vi "SetTempAndMeasure.vi"() -> ()   [LabVIEW 2009]
uses:
  <instrlib>/BK Precision 91xx Series/BK Precision 91xx Series.lvlib
panel:
  out "error out":errorcluster
  in  "Serial Configuration":T1={"Parity(0:none)"=0, "Baud Rate (9600)"=9600, "Data Bits(8)"=8, "Flow Control(None)"=0, " Stop Bits(1.0)"=10} {"Stop Bits(1.0)" items=["1.0"=10, "1.5"=15, "2.0"=20]; "Flow Control(None)" items=["None", "XON/XOFF", "RTS/CTS", "XON/XOFF & RTS/CTS", "DTR/DSR", "XON/XOFF & DTR/DSR"]; "Data Bits(8)" items=["7"=7, "8"=8]; "Baud Rate (9600)" items=["2400"=2400, "4800"=4800, "9600"=9600, "19200"=19200, "38400"=38400]; "Parity(0:none)" items=["None", "Odd", "Even", "Mark", "Space"]}
  in  "VISA resource name":refnum<visa-resource-name>
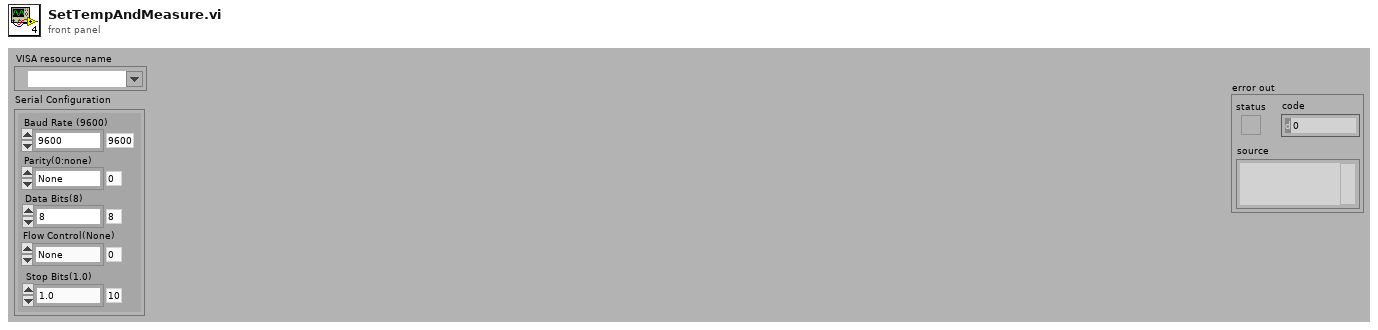
[diagram p1: front panel]
types:
  T1 = cluster{"Parity(0:none)":u16, "Baud Rate (9600)":u16, "Data Bits(8)":u16, "Flow Control(None)":u16, " Stop Bits(1.0)":u16}
  T2 = enum16{"open", "replace", "create", "open or create", "replace or create", "replace or create with confirmation"}
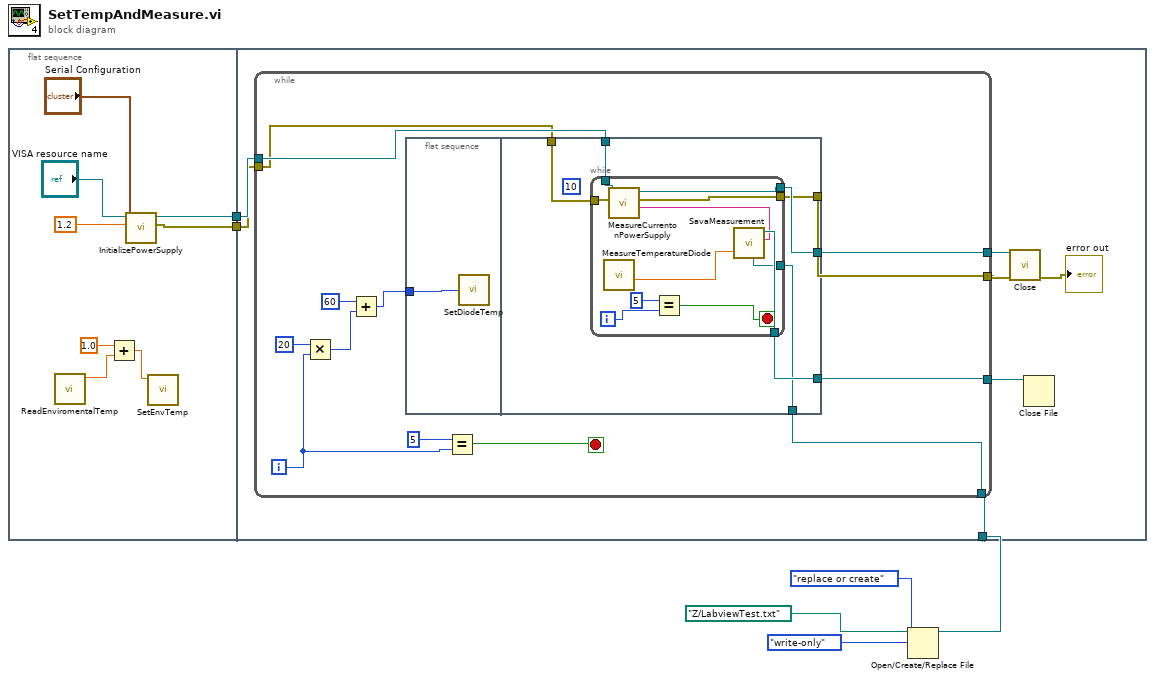
[diagram p0: block diagram]
diagram:
  n1 = flat-sequence {
    tunnel: [w8] -> w2
    tunnel: [w7] -> w1
    tunnel: w3 -> [w17]
    tunnel: w2 -> [w16]
    tunnel: w1 -> [w15]
    frame #0 {
      n2 = call "ReadEnviromentalTemp.vi"() -> ("Probe 1 temperature"=w10:dbl)  [unwired: 10 in, 1 out]
      n3 = Add(x=1.0, y=w10) -> (x+y=w11:dbl)
      n4 = call "InitializePowerSupply.vi"("Serial Configuration"="Serial Configuration", "Manual Range(0.00)"=1.2, "VISA resource name"="VISA resource name") -> ("error out"=w7:errorcluster, "VISA resource name out"=w8:refnum<visa-resource-name>)  [unwired: 7 in]
      n5 = call "SetEnvTemp.vi"("New temperature"=w11) -> ()  [unwired: 10 in, 1 out]
    }
    frame #1 {
      n6 = while {
        tunnel: [w34] -> w20
        tunnel: [w33] -> w19
        tunnel: [w32] -> w18
        tunnel: w17 -> [w31]
        tunnel: w16 -> [w23]
        tunnel: w15 -> [w22]
        i -> [w28]
        stop <- w29 stop-if-true
        n7 = Multiply(x=20, y=w28) -> (x*y=w26:i32)
        n8 = Add(x=60, y=w26) -> (x+y=w24:i32)
        n9 = flat-sequence {
          tunnel: w24 -> [w35]
          tunnel: [w41] -> w34
          tunnel: [w40] -> w33
          tunnel: [w39] -> w32
          tunnel: w31 -> [w38]
          tunnel: w23 -> [w37]
          tunnel: w22 -> [w36]
          frame #0 {
            n10 = call "SetDiodeTemp.vi"(w35) -> ()
          }
          frame #1 {
            (unwired) 10
            n11 = while {
              tunnel: [w52] -> w41
              tunnel: [w51] -> w40
              tunnel: [w50] -> w39
              tunnel: w38 -> [w44]
              tunnel: w37 -> [w43]
              tunnel: w36 -> [w42]
              i -> [w47]
              stop <- w46 stop-if-true
              n12 = call "MeasureTemperatureDiode.vi"() -> ("Celcius"=w49:dbl)  [unwired: 8 in, 3 out]
              n13 = call "MeasureCurrentonPowerSupply.vi"("error in (no error)"=w42, "VISA resource name"=w43) -> ("Measurement"=w48:string, "error out"=w51:errorcluster, "VISA resource name out"=w52:refnum<visa-resource-name>)  [unwired: 7 in]
              n14 = Equal?(x=5, y=w47) -> (x = y?=w46:bool)
              n15 = call "SavaMeasurement.vi"("Measurement"=w48, "refnum out"=w44, "DiodeTemperature"=w49) -> ("refnum out 2"=w50:refnum<file>)  [unwired: 2 in, 1 out]
            }
          }
        }
        n16 = Equal?(x=5, y=w28) -> (x = y?=w29:bool)
      }
      n17 = call <instrlib>:"Close.vi"("error in (no error)"=w19, "VISA resource name"=w20) -> ("error out"=→"error out":errorcluster)  [unwired: 9 in]
      n18 = Close File(refnum=w18) -> ()  [unwired: 1 in, 2 out]
    }
  }
  n19 = Open/Create/Replace File(file path (use dialog)=path "Z:/LabviewTest.txt", operation (0:open)=T2."replace or create", access (0:read/write)=enum16{"read/write", "read-only", "write-only"}."write-only") -> (refnum out=w3:refnum<file>)  [unwired: 3 in, 2 out]
